vi "state_machine.vi"() -> ()   [LabVIEW 2024]
panel:
  out "output waveform":waveform(dbl)
  in  "Pressure sensor":dbl=1.0
  in  "GasX state machine":enum32{"Controls", "Settings"}(tab)
  in  "Fast flush":bool
  out "Waveform Chart":waveform(dbl)(graph)
  in  "GasX ON":bool
  in  "Measure":bool[](array[boolean])=[FALSE, FALSE, FALSE, FALSE]
  in  "Pressure":bool[](array[boolean])=[FALSE, TRUE, FALSE, TRUE]
  in  "Idle":bool[](array[boolean])=[FALSE, FALSE, FALSE, FALSE]
  out "Current state":bool[](array[boolean])
  out "Pressure State OUT":T1(ring)=enum."Measure"
  out "State IN":T1(ring)
  out "Pressure reading":dbl=1.0
  in  "Target pressure":dbl=2.0
  out "Idle State  OUT":T1(ring)
  out "Target pressure reached":bool=TRUE
  in  "Measure pressure":bool
  out "Measure State OUT":T1(ring)
  out "Measure pressure LED":bool
  out "GasX ON LED":bool
  in  "stop 2":bool
  out "Evac State OUT":T1(ring)=enum."Pressure"
  in  "Evac":bool[](array[boolean])=[FALSE, TRUE, TRUE, TRUE]
  in  "GasX":bool[](array[boolean])=[TRUE, TRUE, TRUE, FALSE]
  out "Current state string":string="Idle"
  out "Evac time elapsed (s)":dbl=5.000917911529541 format="%_4g"
  out "GasX time elapsed (s)":dbl=2.0009751319885254 format="%_4g"
  out "GasX State OUT":T1(ring)=enum."Evac"
  out "Pressure time elapsed (s)":dbl format="%_5g"
  out "Measure time elapsed (s)":dbl format="%_5g"
  out "Time":dbl=48.38783264160156 format="%#_4g"
  out "V1":bool
  out "V2":bool
  out "V3":bool
  out "V4":bool
  in  "dt (s)":dbl=1.0
  in  "Pressure State OUT 1":T1(ring)
  in  "Pressure  State OUT 2":T1(ring)=enum."Measure"
  in  "Measure State OUT 1":T1(ring)=enum."Gasx"
  in  "Measure State OUT 2":T1(ring)
  in  "stop":bool
  in  "Idle State  OUT 1":T1(ring)
  in  "Idle State  OUT 2":T1(ring)=enum."Gasx"
  in  "Idle State  OUT 3":T1(ring)=enum."Pressure"
  in  "Evac State OUT 1":T1(ring)=enum."Pressure"
  in  "Evac State OUT 2":T1(ring)=enum."Evac"
  out "Evac current time":timestamp=timestamp(3825219554.041868 s since 1904-01-01)
  out "Evac start time":timestamp=timestamp(3825219549.0409503 s since 1904-01-01)
  out "GasX start time":timestamp
  out "GasX current time":timestamp=timestamp(3825219549.0409503 s since 1904-01-01)
  in  "GasX State OUT 2":T1(ring)=enum."Evac"
  in  "GasX State OUT 1":T1(ring)=enum."Gasx"
  in  "T_measure (s)":dbl
  out "Pressure start time":timestamp
  out "Pressure current time":timestamp
  in  "Pressure State OUT 3":T1(ring)
  out "Measure start time":timestamp
  out "Measure current time":timestamp
  in  "Measure State OUT3":T1(ring)=enum."Gasx"
  in  "T_flush (s)":dbl
  in  "T_evac (s)":dbl
  in  "T_pressure (s)":dbl
  out "Pressure start time (from Idle) (s)":timestamp
  in  "While loop wait (ms)":u32=100
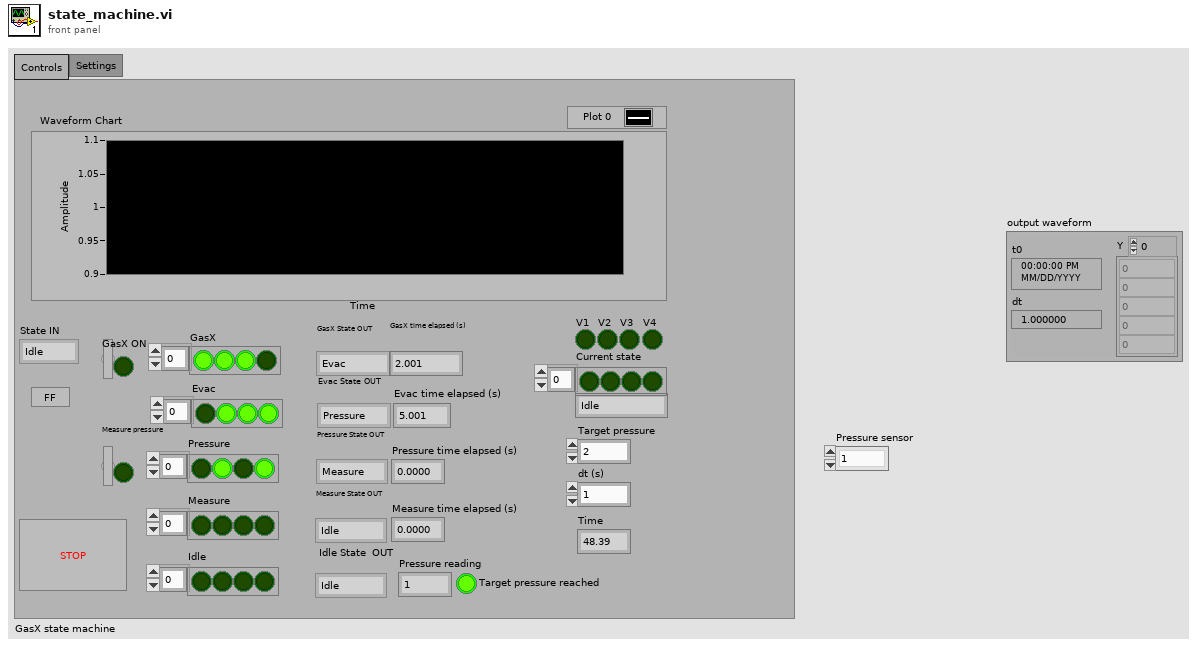
[diagram p1: front panel]
types:
  T1 = enum16{"Idle", "Gasx", "Evac", "Pressure", "Measure"}
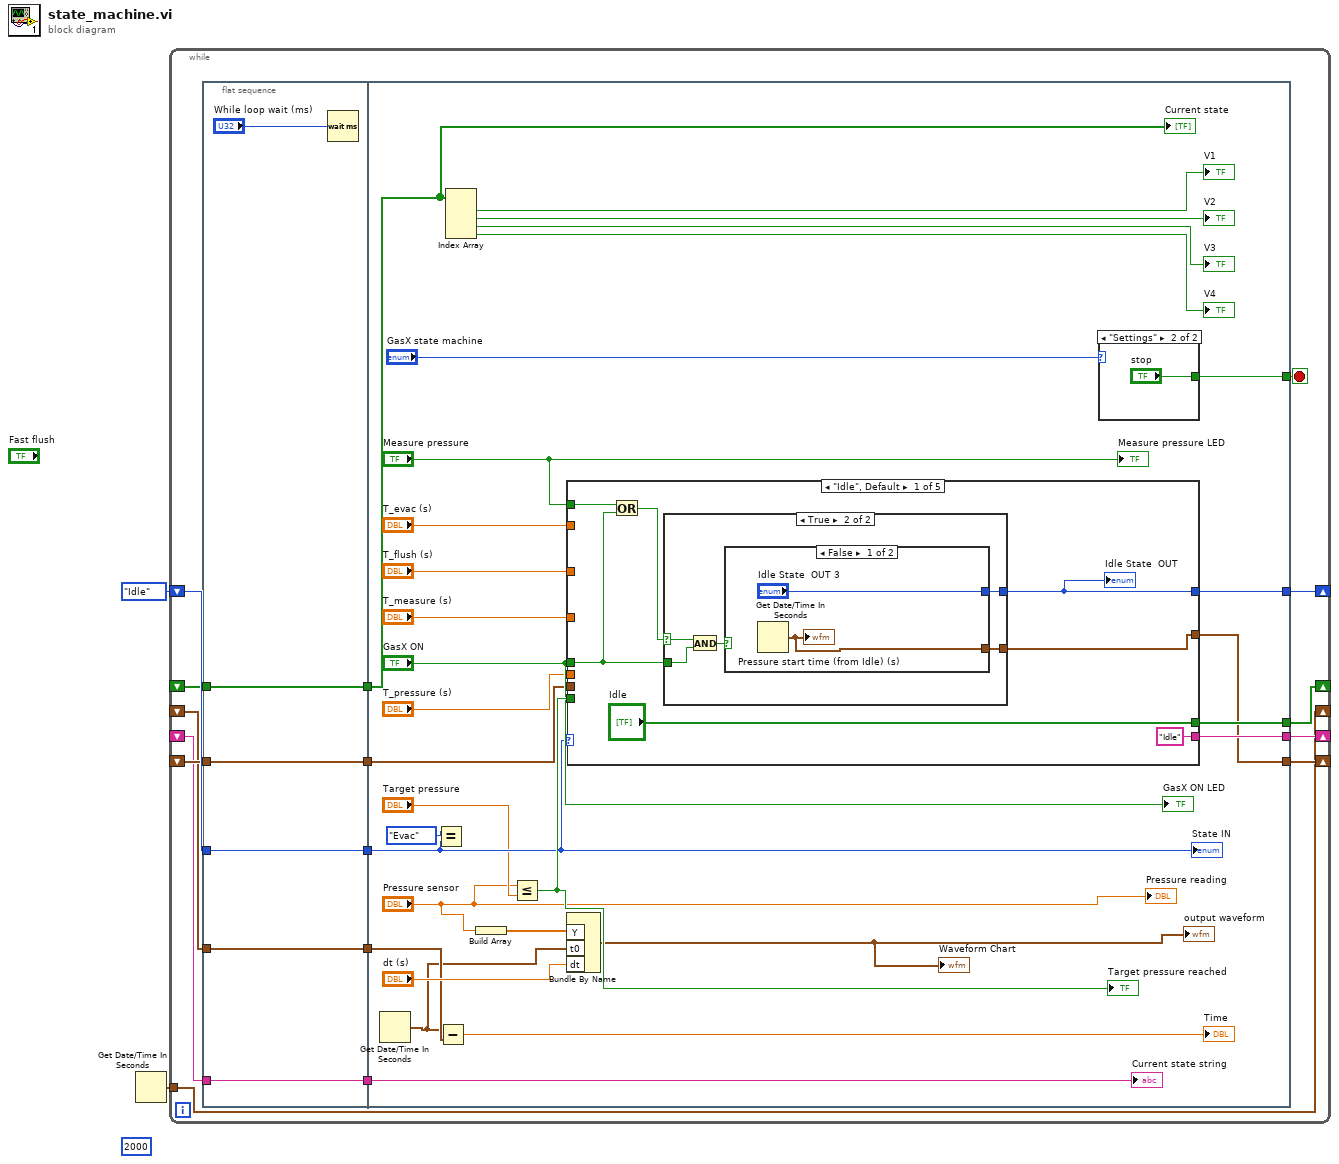
[diagram p0: block diagram]
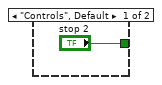
[diagram p2: hidden frame]
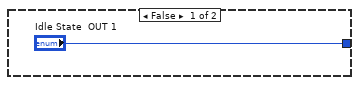
[diagram p3: hidden frame]
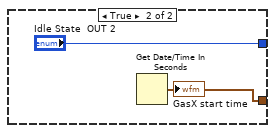
[diagram p4: hidden frame]
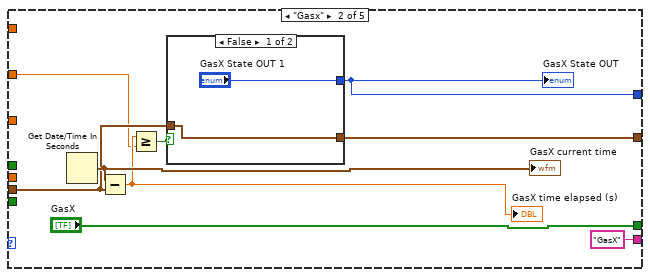
[diagram p5: hidden frame]
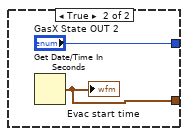
[diagram p6: hidden frame]
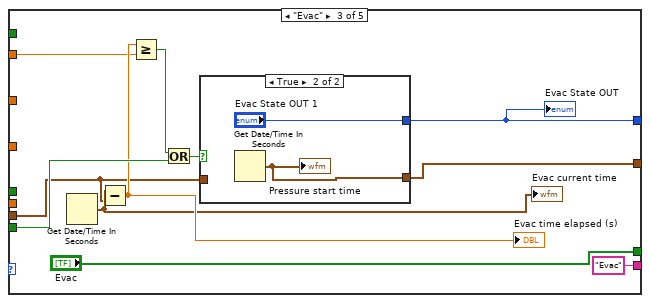
[diagram p7: hidden frame]
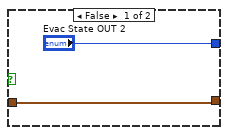
[diagram p8: hidden frame]
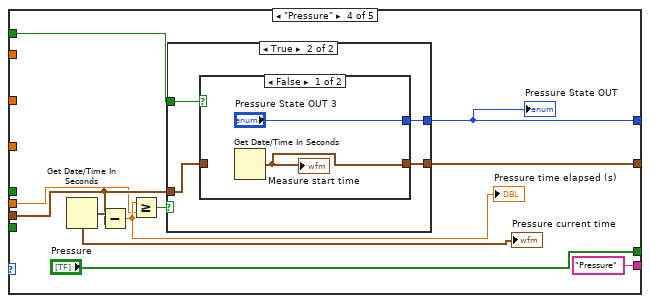
[diagram p9: hidden frame]
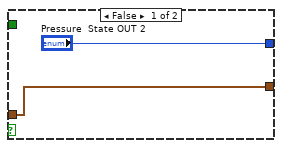
[diagram p10: hidden frame]
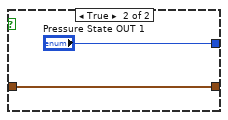
[diagram p11: hidden frame]
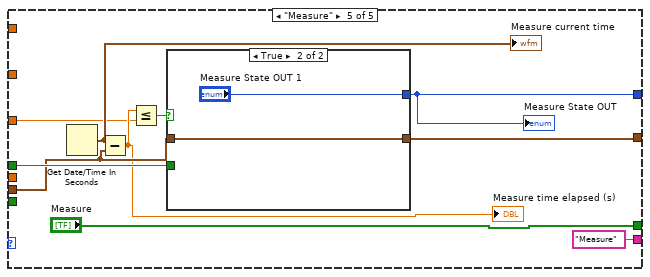
[diagram p12: hidden frame]
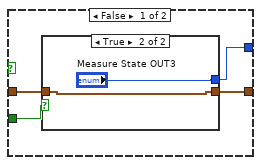
[diagram p13: hidden frame]
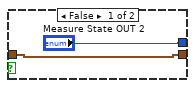
[diagram p14: hidden frame]
diagram:
  (unwired) u32 2000 ("Timer start 2")
  n1 = Get Date/Time In Seconds() -> (seconds since 1Jan1904=w1:timestamp)
  n2 = while {
    shift-right: [w18] -> _
    shift-left: T1."Idle" ("Measure State OUT 1") -> [w16]
    shift-right: [w10] -> _
    shift-left: _ -> [w15]
    shift-right: [w14] -> _
    shift-left: _ -> [w13]
    shift-right: [w12] -> _
    shift-left: _ -> [w11]
    tunnel: w1 -> [w9]
    shift-right: [w9] -> _
    shift-left: _ -> [w8]
    stop <- w17 stop-if-true
    n3 = flat-sequence {
      tunnel: w8 -> [w20]
      tunnel: w11 -> [w21]
      tunnel: w13 -> [w22]
      tunnel: w15 -> [w23]
      tunnel: w16 -> [w24]
      tunnel: [w24] -> w7
      tunnel: [w23] -> w6
      tunnel: [w22] -> w5
      tunnel: [w21] -> w4
      tunnel: [w20] -> w3
      tunnel: [w54] -> w18
      tunnel: [w50] -> w17
      tunnel: [w44] -> w14
      tunnel: [w43] -> w12
      tunnel: [w41] -> w10
      tunnel: w7 -> [w47]
      tunnel: w6 -> [w45]
      tunnel: w5 -> [w36]
      tunnel: w4 -> [w42]
      tunnel: w3 -> [w28]
      frame #0 {
        n4 = Wait (ms)(milliseconds to wait="While loop wait (ms)") -> ()  [unwired: 1 out]
      }
      frame #1 {
        n5 = Get Date/Time In Seconds() -> (seconds since 1Jan1904=w25:timestamp)
        n6 = Equal?(x=T1."Evac" ("State IN"), y=w47) -> ()  [unwired: 1 out]
        n7 = Subtract(x=w25, y=w28) -> (x-y=→"Time":dbl)
        n8 = Index Array(array=w36) -> (element #1=→"V1":bool, element #2=→"V2":bool, element #3=→"V3":bool, element #4=→"V4":bool)  [unwired: 4 in]
        n9 = Build Array("Pressure sensor") -> (w30:dbl[])
        n10 = Less Or Equal?(x="Pressure sensor", y="Target pressure") -> (x <= y?=w53:bool)
        "Target pressure reached" <- w53
        n11 = case shown="\"Idle\", Default" w47 {
          tunnel: [w59 w82 w97 w111 w131] -> w54
          tunnel: w53 -> [_ _ w96 _ _]
          tunnel: "Measure pressure" -> [w63 _ _ w103 _]
          tunnel: "GasX ON" -> [w60 _ _ _ w127]
          tunnel: "T_measure (s)" -> [_ _ _ _ w122]
          tunnel: [w57 w76 w88 w105 w125] -> w41
          tunnel: w45 -> [_ w75 w89 w106 w126]
          tunnel: ["Idle" "GasX" "Evac" "Pressure" "Measure"] -> w43
          tunnel: ["Idle" "GasX" "Evac" "Pressure" "Measure"] -> w44
          tunnel: "T_flush (s)" -> [_ w74 _ _ _]
          tunnel: "T_evac (s)" -> [_ _ w87 _ _]
          tunnel: "T_pressure (s)" -> [_ _ _ w102 _]
          frame "Idle", Default {
            n12 = Or(x=w63, y=w60) -> (x .or. y?=w61:bool)
            n13 = case shown="True" w61 {
              selector: w61 -> [_ w68]
              tunnel: ["Idle State  OUT 1" w69] -> w59
              tunnel: w60 -> [_ w67]
              tunnel: [_ w65] -> w57
              frame False {
              }
              frame True {
                n14 = And(x=w68, y=w67) -> (x .and. y?=w66:bool)
                n15 = case shown="False" w66 {
                  tunnel: ["Idle State  OUT 3" "Idle State  OUT 2"] -> w69
                  tunnel: [w70 w72] -> w65
                  frame False {
                    n16 = Get Date/Time In Seconds() -> (seconds since 1Jan1904=w70:timestamp)
                    "Pressure start time (from Idle) (s)" <- w70
                  }
                  frame True {
                    n17 = Get Date/Time In Seconds() -> (seconds since 1Jan1904=w72:timestamp)
                    "GasX start time" <- w72
                  }
                }
              }
            }
            "Idle State  OUT" <- w59
          }
          frame "Gasx" {
            n18 = Get Date/Time In Seconds() -> (seconds since 1Jan1904=w79:timestamp)
            "GasX current time" <- w79
            n19 = Subtract(x=w79, y=w75) -> (x-y=w78:dbl)
            "GasX time elapsed (s)" <- w78
            n20 = Greater Or Equal?(x=w78, y=w74) -> (x >= y?=w77:bool)
            n21 = case shown="False" w77 {
              tunnel: ["GasX State OUT 1" "GasX State OUT 2"] -> w82
              tunnel: [w83 w85] -> w76
              tunnel: w75 -> [w83 _]
              frame False {
              }
              frame True {
                n22 = Get Date/Time In Seconds() -> (seconds since 1Jan1904=w85:timestamp)
                "Evac start time" <- w85
              }
            }
            "GasX State OUT" <- w82
          }
          frame "Evac" {
            n23 = Get Date/Time In Seconds() -> (seconds since 1Jan1904=w92:timestamp)
            "Evac current time" <- w92
            n24 = Subtract(x=w92, y=w89) -> (x-y=w93:dbl)
            "Evac time elapsed (s)" <- w93
            n25 = Greater Or Equal?(x=w93, y=w87) -> (x >= y?=w95:bool)
            n26 = Or(x=w95, y=w96) -> (x .or. y?=w94:bool)
            n27 = case shown="True" w94 {
              tunnel: ["Evac State OUT 2" "Evac State OUT 1"] -> w97
              tunnel: w89 -> [w98 _]
              tunnel: [w98 w100] -> w88
              frame False {
              }
              frame True {
                n28 = Get Date/Time In Seconds() -> (seconds since 1Jan1904=w100:timestamp)
                "Pressure start time" <- w100
              }
            }
            "Evac State OUT" <- w97
          }
          frame "Pressure" {
            n29 = Get Date/Time In Seconds() -> (seconds since 1Jan1904=w108:timestamp)
            "Pressure current time" <- w108
            n30 = Subtract(x=w108, y=w106) -> (x-y=w107:dbl)
            "Pressure time elapsed (s)" <- w107
            n31 = Greater Or Equal?(x=w107, y=w102) -> (x >= y?=w104:bool)
            n32 = case shown="True" w104 {
              tunnel: ["Pressure  State OUT 2" w117] -> w111
              tunnel: w106 -> [w112 w115]
              tunnel: [w112 w114] -> w105
              tunnel: w103 -> [_ w116]
              frame False {
              }
              frame True {
                n33 = case shown="False" w116 {
                  tunnel: ["Pressure State OUT 3" "Pressure State OUT 1"] -> w117
                  tunnel: w115 -> [_ w120]
                  tunnel: [w118 w120] -> w114
                  frame False {
                    n34 = Get Date/Time In Seconds() -> (seconds since 1Jan1904=w118:timestamp)
                    "Measure start time" <- w118
                  }
                  frame True {
                  }
                }
              }
            }
            "Pressure State OUT" <- w111
          }
          frame "Measure" {
            n35 = Get Date/Time In Seconds() -> (seconds since 1Jan1904=w128:timestamp)
            "Measure current time" <- w128
            n36 = Subtract(x=w128, y=w126) -> (x-y=w123:dbl)
            "Measure time elapsed (s)" <- w123
            n37 = Less Or Equal?(x=w123, y=w122) -> (x <= y?=w124:bool)
            n38 = case shown="True" w124 {
              tunnel: [w134 "Measure State OUT 1"] -> w131
              tunnel: w127 -> [w135 _]
              tunnel: w126 -> [w133 w140]
              tunnel: [w132 w140] -> w125
              frame False {
                n39 = case shown="True" w135 {
                  tunnel: ["Measure State OUT 2" "Measure State OUT3"] -> w134
                  tunnel: w133 -> [w136 w138]
                  tunnel: [w136 w138] -> w132
                  frame False {
                  }
                  frame True {
                  }
                }
              }
              frame True {
              }
            }
            "Measure State OUT" <- w131
          }
        }
        n40 = Bundle By Name("Y"=w30, "t0"=w25, "dt"="dt (s)") -> (→"output waveform" →"Waveform Chart":waveform(dbl))  [unwired: 1 in]
        n41 = case shown="\"Settings\"" "GasX state machine" {
          tunnel: ["stop 2" "stop"] -> w50
          frame "Controls", Default {
          }
          frame "Settings" {
          }
        }
        "State IN" <- w47
        "Pressure reading" <- "Pressure sensor"
        "Measure pressure LED" <- "Measure pressure"
        "GasX ON LED" <- "GasX ON"
        "Current state" <- w36
        "Current state string" <- w42
      }
    }
  }
